vi "Legend0002.vi"   [LabVIEW 2013]
uses:
  <vilib>/Heliosphere Research LLC/Advanced Plotting Toolkit/api_plotting/Histogram_Automatic.vi
  <vilib>/Heliosphere Research LLC/Advanced Plotting Toolkit/Advanced Plotting Toolkit.lvlib
types:
  T1 = typedef "Advanced Plotting Toolkit.lvlib/PlotID.ctl" = i32
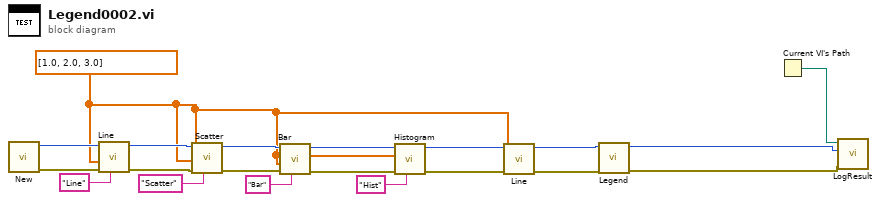
[diagram p0: block diagram]
diagram:
  w1 = dbl[] [1.0, 2.0, 3.0] ("Y Data")
  n1 = call <vilib>:"New.vi"() -> ("error out"=w15:errorcluster, "Plot ID"=w19:T1)  [unwired: 10 in]
  n2 = call <vilib>:"Line.vi"("Legend Title"="Line", "error in (no error)"=w15, "Y Data"=w1, "Plot ID"=w19) -> ("error out"=w14:errorcluster, "Plot ID out"=w18:T1)  [unwired: 6 in]
  n3 = call <vilib>:"Scatter.vi"("Legend Title"="Scatter", "error in (no error)"=w14, "Y Data"=w1, "X Data"=w1, "Plot ID"=w18) -> ("error out"=w13:errorcluster, "Plot ID Out"=w17:T1)  [unwired: 5 in]
  n4 = call <vilib>:"Bar.vi"("Legend Title"="Bar", "error in (no error)"=w13, "Bar Lengths"=w1, "Plot ID"=w17) -> ("error out"=w12:errorcluster, "Plot ID Out"=w16:T1)  [unwired: 6 in]
  n5 = call-poly <vilib>:"Histogram.vi"("Legend Title"="Hist", "error in (no error)"=w12, "Data"=w1, "Plot ID"=w16) -> ("error out"=w4:errorcluster, "Plot ID Out"=w7:T1)  [unwired: 6 in]
  n6 = call <vilib>:"Line.vi"("error in (no error)"=w4, "Y Data"=w1, "Plot ID"=w7) -> ("error out"=w3:errorcluster, "Plot ID out"=w6:T1)  [unwired: 7 in]
  n7 = call <vilib>:"Legend.vi"("error in (no error)"=w3, "Plot ID"=w6) -> ("error out"=w2:errorcluster, "Plot ID Out"=w5:T1)  [unwired: 8 in]
  n8 = Current VI's Path() -> (path=w20:path)
  n9 = call "LogResult.vi"("Test Result"=w2, "Test Artifact"=w5, "VI Path"=w20) -> ()  [unwired: 9 in]
